vi "Packet_decode_Transform3d.vi"(7 "NextByte in":i32, 9 "RawData":u8[](array[numeric])) -> (1 "NextByte out":i32, 3 "Transform3d":T1 {"TRANSLATION3D"."Z" format="%14.3f"; "TRANSLATION3D"."Y" format="%14.3f"; "TRANSLATION3D"."X" format="%14.3f"})   [LabVIEW 2019, in "PhotonVisionLib.lvlib"]
uses:
  PhotonVisionLib.lvlib
  <vilib>/Rock Robotics/WPI/ThirdParty/JAS_Junk/TrajLib/TypeDef/TRANSFORM3D.ctl
  <vilib>/Rock Robotics/WPI/ThirdParty/JAS_Junk/TrajLib/TypeDef/TRANSLATION3D.ctl
  <vilib>/Rock Robotics/WPI/ThirdParty/JAS_Junk/TrajLib/TypeDef/ROTATION3D.ctl
  <vilib>/Rock Robotics/WPI/ThirdParty/JAS_Junk/TrajLib/TypeDef/QUATERNION.ctl
  <vilib>/Rock Robotics/WPI/ThirdParty/JAS_Junk/TrajLib/VI/Quaternion_Normalize.vi
  <vilib>/Rock Robotics/WPI/ThirdParty/JAS_Junk/TrajLib/VI/Quaternion_New_Default.vi
  <vilib>/Rock Robotics/WPI/ThirdParty/JAS_Junk/TrajLib/Trajectory_Library.lvlib
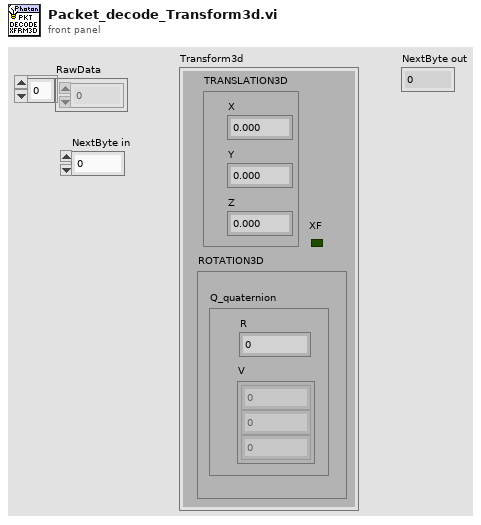
[diagram p1: front panel]
types:
  T1 = typedef "Trajectory_Library.lvlib/TRANSFORM3D.ctl" = cluster{"TRANSLATION3D":T2, "ROTATION3D":T3, "XF":bool}
  T2 = typedef "Trajectory_Library.lvlib/TRANSLATION3D.ctl" = cluster{"X":dbl, "Y":dbl, "Z":dbl}
  T3 = typedef "Trajectory_Library.lvlib/ROTATION3D.ctl" = cluster{"Q_quaternion":T4}
  T4 = typedef "Trajectory_Library.lvlib/QUATERNION.ctl" = cluster{"R":dbl, "V":dbl[]}
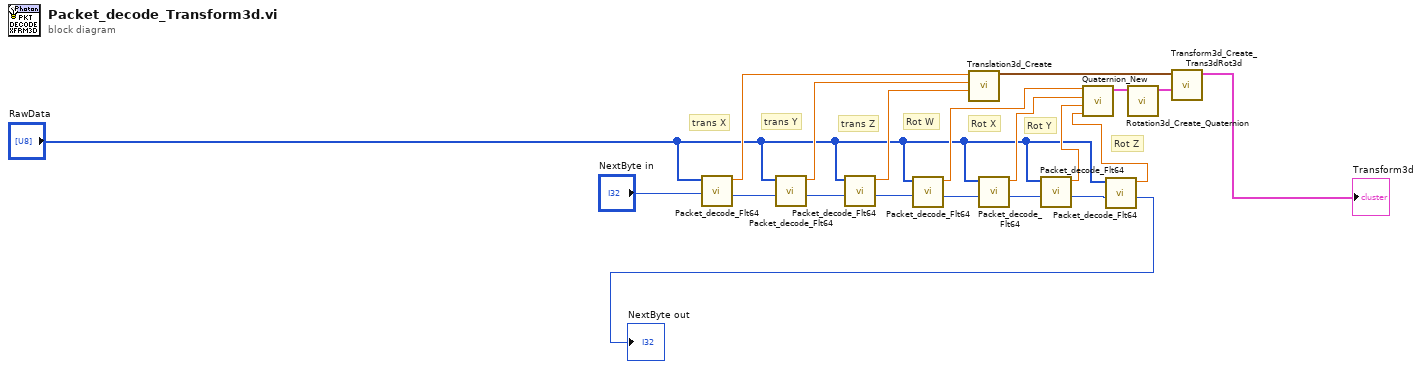
[diagram p0: block diagram]
diagram:
  # "Rot Z"
  # "Rot Y"
  # "Rot X"
  # "Rot W"
  # "trans Z"
  # "trans Y"
  # "trans X"
  n1 = call "Packet_decode_Flt64.vi"("StartByte"="NextByte in", "RawData"="RawData") -> ("NextByte"=w1:i32, "Flt64_Value"=w9:dbl)  [unwired: 8 in]
  n2 = call "Packet_decode_Flt64.vi"("StartByte"=w1, "RawData"="RawData") -> ("NextByte"=w2:i32, "Flt64_Value"=w10:dbl)  [unwired: 8 in]
  n3 = call "Packet_decode_Flt64.vi"("StartByte"=w2, "RawData"="RawData") -> ("NextByte"=w7:i32, "Flt64_Value"=w11:dbl)  [unwired: 8 in]
  n4 = call "Packet_decode_Flt64.vi"("StartByte"=w7, "RawData"="RawData") -> ("NextByte"=w4:i32, "Flt64_Value"=w16:dbl)  [unwired: 8 in]
  n5 = call <vilib>:"Translation3d_Create.vi"("Z"=w11, "Y"=w10, "X"=w9) -> ("TRANSLATION3D"=w12:T2)  [unwired: 8 in]
  n6 = call "Packet_decode_Flt64.vi"("StartByte"=w4, "RawData"="RawData") -> ("NextByte"=w5:i32, "Flt64_Value"=w17:dbl)  [unwired: 8 in]
  n7 = call "Packet_decode_Flt64.vi"("StartByte"=w5, "RawData"="RawData") -> ("NextByte"=w6:i32, "Flt64_Value"=w18:dbl)  [unwired: 8 in]
  n8 = call "Packet_decode_Flt64.vi"("StartByte"=w6, "RawData"="RawData") -> ("NextByte"=→"NextByte out":i32, "Flt64_Value"=w19:dbl)  [unwired: 8 in]
  n9 = call <vilib>:"Quaternion_New.vi"("Z"=w19, "Y"=w18, "X"=w17, "W"=w16) -> ("out Quaternion"=w15:T4)  [unwired: 7 in]
  n10 = call <vilib>:"Rotation3d_Create_Quaternion.vi"("Quaternion"=w15) -> ("Rotation3d"=w13:T3)  [unwired: 10 in]
  n11 = call <vilib>:"Transform3d_Create_Trans3dRot3d.vi"("Rotation3d"=w13, "Translation3d"=w12) -> ("Transform3d"=→"Transform3d":T1)  [unwired: 9 in]
